vi "readLogAirStatus.vi"(8 "error in (no error)":errorcluster, 10 "Parser":refnum<class "U8ArrayParserAutoIndexing.lvclass">, 11 "M1M3SAL in":refnum<class "M1M3SAL.lvclass">) -> (0 "error out":errorcluster, 2 "EventAirStatus":variant, 3 "M1M3SAL out":refnum<class "M1M3SAL.lvclass">)   [LabVIEW 2016, in "M1M3SupportCommunicator.lvlib" / "M1M3SAL.lvclass"]
uses:
  M1M3SAL.lvclass
  Common_RT_Utilities/U8ArrayParserAutoIndexing/U8ArrayParserAutoIndexing.lvclass
  DataTypes/Topics/EventAirStatus.ctl
  DataTypes/Topics/Parts/Timestamp.ctl
  DataTypes/Topics/M1M3SupportTopics.lvlib
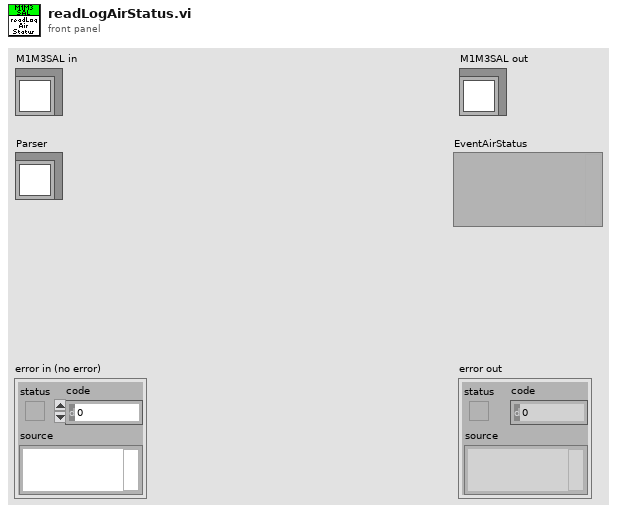
[diagram p1: front panel]
types:
  T1 = typedef "M1M3SupportTopics.lvlib/EventAirStatus.ctl" = cluster{"Timestamp":T2, "AirCommandedOn":bool, "AirOn":bool, "AirPressureOk":bool, "HardpointAirPressureOk":bool}
  T2 = typedef "M1M3SupportTopics.lvlib/Timestamp.ctl" = dbl
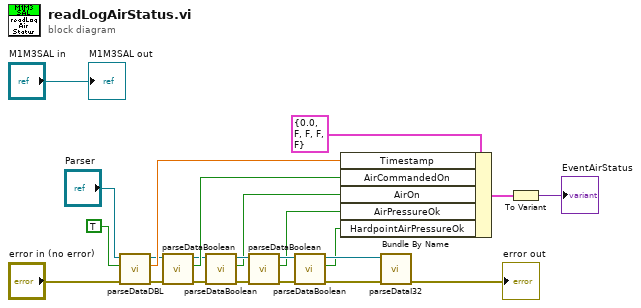
[diagram p0: block diagram]
diagram:
  n1 = call "parseDataDBL.vi"("error in (no error)"="error in (no error)", "OverrideSwapBytes"=TRUE, "U8ArrayParserAutoIndexing in"="Parser") -> ("error out"=w13:errorcluster, "Data"=w16:dbl, "U8ArrayParserAutoIndexing out"=w15:refnum<class "U8ArrayParserAutoIndexing.lvclass">)  [unwired: 6 in]
  n2 = call "parseDataBoolean.vi"("error in (no error)"=w13, "U8ArrayParserAutoIndexing in"=w15) -> ("error out"=w11:errorcluster, "Data"=w14:bool, "U8ArrayParserAutoIndexing out"=w10:refnum<class "U8ArrayParserAutoIndexing.lvclass">)  [unwired: 7 in]
  n3 = call "parseDataBoolean.vi"("error in (no error)"=w11, "U8ArrayParserAutoIndexing in"=w10) -> ("error out"=w4:errorcluster, "Data"=w3:bool, "U8ArrayParserAutoIndexing out"=w9:refnum<class "U8ArrayParserAutoIndexing.lvclass">)  [unwired: 7 in]
  n4 = call "parseDataBoolean.vi"("error in (no error)"=w4, "U8ArrayParserAutoIndexing in"=w9) -> ("error out"=w5:errorcluster, "Data"=w2:bool, "U8ArrayParserAutoIndexing out"=w8:refnum<class "U8ArrayParserAutoIndexing.lvclass">)  [unwired: 7 in]
  n5 = call "parseDataBoolean.vi"("error in (no error)"=w5, "U8ArrayParserAutoIndexing in"=w8) -> ("error out"=w6:errorcluster, "Data"=w1:bool, "U8ArrayParserAutoIndexing out"=w7:refnum<class "U8ArrayParserAutoIndexing.lvclass">)  [unwired: 7 in]
  n6 = Bundle By Name(cluster=T1 {"Timestamp"=0.0, "AirCommandedOn"=FALSE, "AirOn"=FALSE, "AirPressureOk"=FALSE, "HardpointAirPressureOk"=FALSE} ("EventAirStatus"), "Timestamp"=w16, "AirCommandedOn"=w14, "AirOn"=w3, "AirPressureOk"=w2, "HardpointAirPressureOk"=w1) -> (w22:T1)
  n7 = call "parseDataI32.vi"("error in (no error)"=w6, "U8ArrayParserAutoIndexing in"=w7) -> ("error out"=→"error out":errorcluster)  [unwired: 7 in, 2 out]
  n8 = To Variant(anything=w22) -> (Variant=→"EventAirStatus":variant)
  "M1M3SAL out" <- "M1M3SAL in"
